vi "Stop Core.vi"(10 "final error code":i32, 11 "System in":refnum<class "System.lvclass">) -> (3 "System out":refnum<class "System.lvclass">)   [LabVIEW 2013, in "System.lvlib" / "System.lvclass"]
doc: "(<B>Filename</B>: Actor Framework.lvlib:Actor.lvclass:Stop Core.vi)\n\nDefines what the actor does before it stops. Use the <B>final error code</B> input to determine whether the actor shut down in response to an error.\n\nBy default, this method does nothing. A descendant class may override it to define behavior, such as shutting down any processes the actor initiated in its override of the Actor Core method."
uses:
  System.lvclass
  <vilib>/ni/Actors/State Actor/State Actor/State Actor.lvclass
  System.lvclass/System.ctl
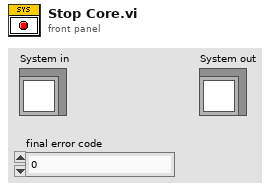
[diagram p1: front panel]
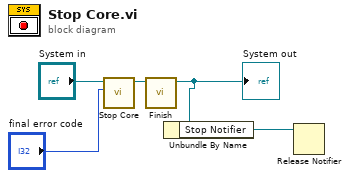
[diagram p0: block diagram]
diagram:
  n1 = call-parent "Stop Core.vi"("final error code"="final error code", "Actor in"="System in") -> ("Actor out"=w4:refnum<class "System.lvclass">)  [unwired: 9 in]
  n2 = call-dynamic "Finish.vi"("System in"=w4) -> ("System out"=w2:refnum<class "System.lvclass">)  [unwired: 9 in, 1 out]
  "System out" <- w2
  n3 = Unbundle By Name(w2) -> ("Stop Notifier"=w1:refnum<notifier>)
  n4 = Release Notifier(notifier=w1) -> ()  [unwired: 2 in, 3 out]
